vi "Distance Calculation.vi"(8 "n":dbl, 10 "PLm":dbl, 11 "PL":dbl) -> (2 "d":dbl)   [LabVIEW 2026]
uses:
  <vilib>/express/express arith-compare/Formula/XNode/ExpressFormulaBlockNode.xnode
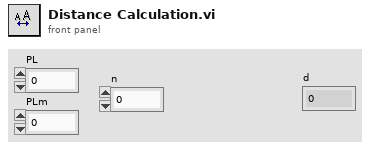
[diagram p1: front panel]
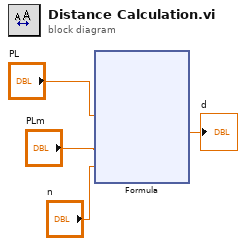
[diagram p0: block diagram]
diagram:
  n1 = xnode "Formula"("PL"="PL", "PLm"="PLm", "n"="n") -> ("Result"=→"d":dbl)  [unwired: 1 in, 1 out]
